vi "UE9 Stream Example LJ_swNONE.vi"() -> ()   [LabVIEW 2021]
panel:
  out "UD Backlog [%]":dbl format="%.2f"
  in  "AIN Range":u16(ring) items=["LJ_rgBIP5V", "LJ_rgUNI5V", "LJ_rgUNI2P5V", "LJ_rgUNI1P25V", "LJ_rgUNIP625V"]
  out "Actual Scan Rate (Hz)":dbl=1000.0 format="%.3f"
  out "ms Per Loop":u32
  out "Comm Backlog":dbl format="%.2f"
  out "Scans Retrieved Sec (measured)":dbl format="%.2f"
  out "# Scans Read":i32
  out "# of iterations":i32
  out "Data":dbl[][](array[numeric]) format="%.3f"
  in  "Scan Rate (Hz)":dbl=1000.0 format="%.3f"
  in  "Scan List":u8[](array[numeric])=[0, 1, 2, 3]
  in  "Data File Extension":string="dat"
  out "Current Data File":path
  in  "Data File Prefix":string="data"
  in  "Write To File":bool
  in  "FirstFound":bool=TRUE
  in  "stop":bool
  in  "ConnectionType":u16(ring) items=["LJ_ctUSB", "LJ_ctETHERNET"]
  in  "Address":string="192.168.1.209"
  out "Error Message":string
  in  "Resolution":i32=12
  # "The actual scans/sec is controlled\nby hardware and is known.  This\n\"measured\" suggests the rate at\nwhich data is being retreived."
  # "Specify an IP address for Ethernet, or Local ID\nfor USB.  If FirstFound is selected, Local ID is\nignored for USB.  Clear FirstFound if using Ethernet."
  # "(for all channels)"
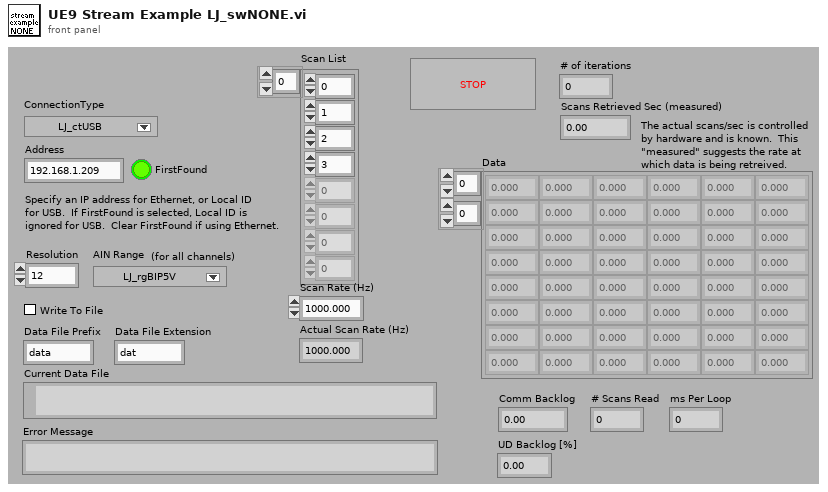
[diagram p1: front panel]
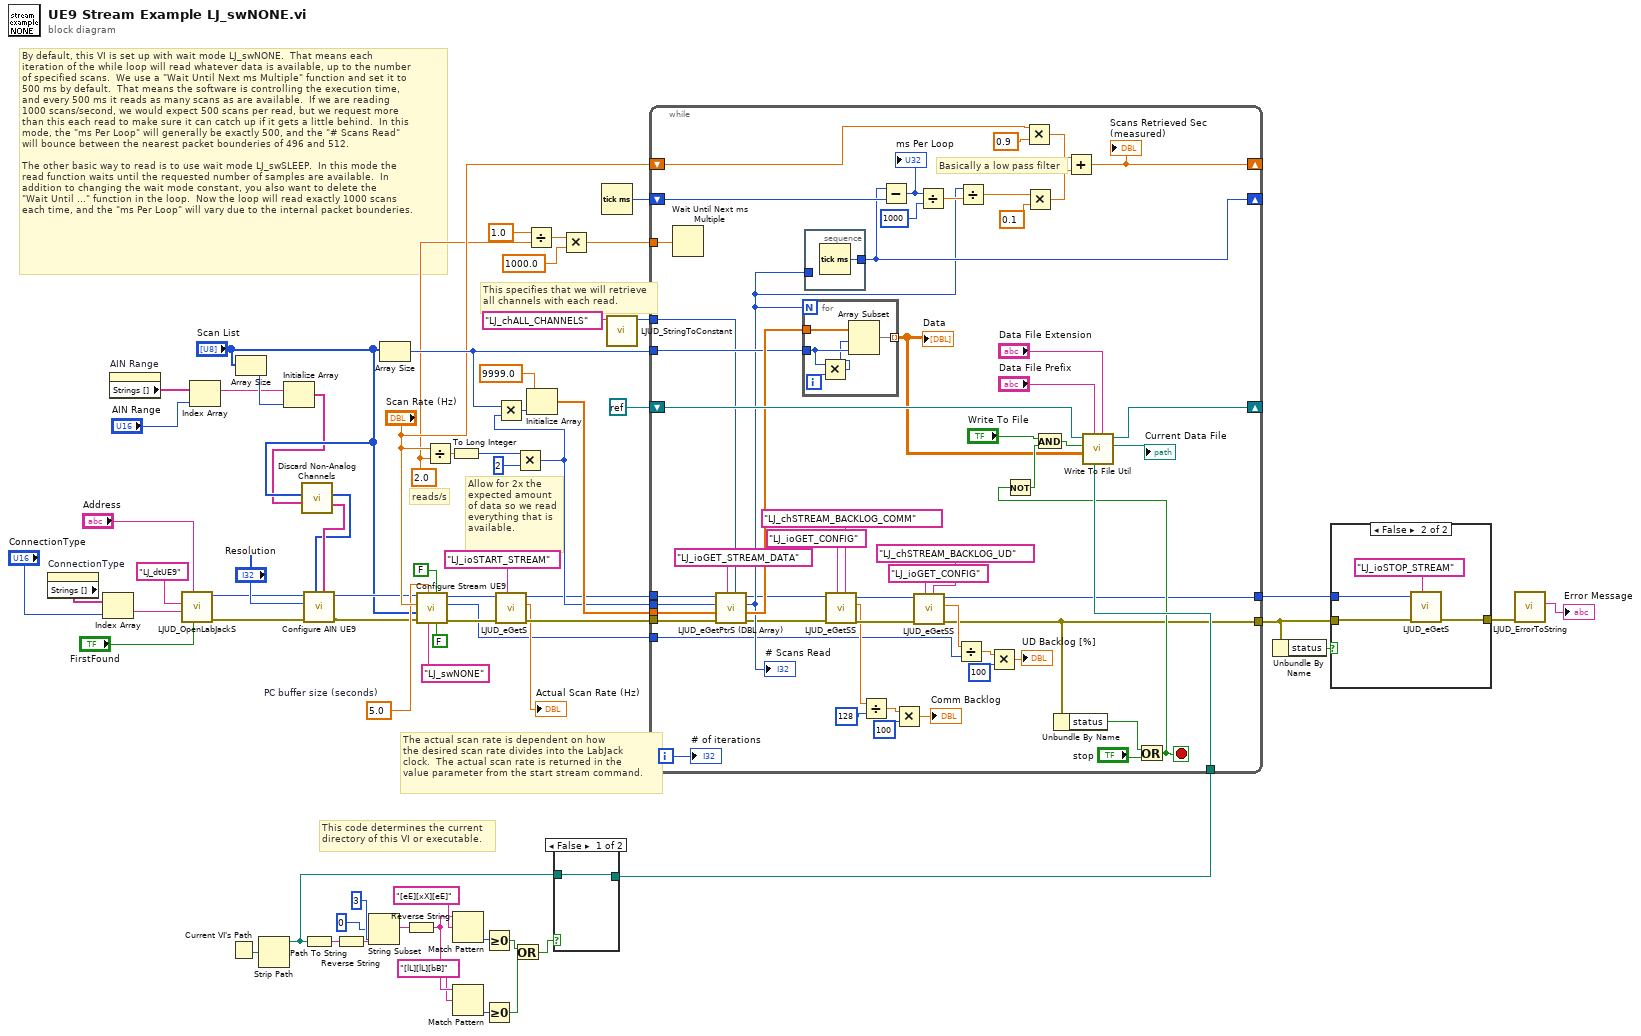
[diagram p0: block diagram]
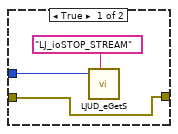
[diagram p2: hidden frame]
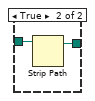
[diagram p3: hidden frame]
diagram:
  w30 = 5.0  # PC buffer size (seconds)
  w37 = 2.0 ("y")
  # "This specifies that we will retrieve\nall channels with each read."
  # "The actual scan rate is dependent on how\nthe desired scan rate divides into the LabJack\nclock.  The actual scan rate is returned in the\nvalue parameter from the start stream command."
  # "By default, this VI is set up with wait mode LJ_swNONE.  That means each\niteration of the while loop will read whatever data is available, up to the number\nof specified scans.  We use a \"Wait Until Next ms Multiple\" function and set it to\n500 ms by default.  That means the software is controlling the execution time,\nand every 500 ms it reads as many scans as are available.  If we are reading\n1000 scans/second, we would expect 500 scans per read, but we request more\nthan this each read to make sure it can catch up if it gets a little behind.  In this\nmode, the \"ms Per Loop\" will generally be exactly 500, and the \"# Scans Read\"\nwill bounce between the nearest packet bounderies of 496 and 512.\n\nThe other basic way to read is to use wait mode LJ_swSLEEP.  In this mode the\nread function waits until the requested number of samples are available.  In\naddition to changing the wait mode constant, you also want to delete the\n\"Wait Until ...\" function in the loop.  Now the loop will read exactly 1000 scans\neach time, and the \"ms Per Loop\" will vary due to the internal packet bounderies."
  # "reads/s"
  # "Allow for 2x the\nexpected amount\nof data so we read\neverything that is\navailable."
  # "This code determines the current\ndirectory of this VI or executable."
  n1 = property on="ConnectionType" class="Ring (strict)"() -> ("Strings []"=w12:string[])  [unwired: 2 in, 2 out]
  n2 = Index Array(array=w12, index="ConnectionType") -> (element=w10:string)
  n3 = property on="AIN Range" class="Ring (strict)"() -> ("Strings []"=w20:string[])  [unwired: 2 in, 2 out]
  n4 = call "LJUD_OpenLabJackS.vi"("FirstFound"="FirstFound", "Address"="Address", "ConnectionType"=w10, "DeviceType"="LJ_dtUE9") -> ("error out"=w16:errorcluster, "Handle"=w17:i32)  [unwired: 5 in, 1 out]
  n5 = Index Array(array=w20, index="AIN Range") -> (element=w18:string)
  n6 = Current VI's Path() -> (path=w68:path)
  n7 = Array Size(array="Scan List") -> (size(s)=w23:i32)
  n8 = Strip Path(path=w68) -> (stripped path=w60:path)  [unwired: 1 out]
  n9 = Initialize Array(w18, w23) -> (w4:string[])
  n10 = call "Discard Non-Analog Channels.vi"("Ranges In"=w4, "Channels In"="Scan List") -> ("Ranges Out"=w3:string[], "Channels Out"=w2:i32[])  [unwired: 6 in, 2 out]
  n11 = call "Configure AIN UE9.vi"("Ranges"=w3, "Channels"=w2, "error in"=w16, "Resolution"="Resolution", "Handle In"=w17) -> ("error out"=w26:errorcluster, "Handle Out"=w25:i32)  [unwired: 5 in]
  n12 = Path To String(path=w60) -> (string=w67:string)
  n13 = Reverse String(1:w67) -> (0:w66:string)
  n14 = String Subset(string=w66, offset (0)=0, length (rest)=3 ("length")) -> (substring=w63:string)
  n15 = Array Size(array="Scan List") -> (size(s)=w44:i32)
  n16 = Reverse String(1:w63) -> (0:w59:string)
  n17 = call "Configure Stream UE9.vi"("External Scan Trigger"=FALSE, "Scan Clock Output"=FALSE, "Wait Mode"="LJ_swNONE" ("Wait Mode (2)"), "PC buffer size (seconds)"=w30, "error in"=w26, "Scan List"="Scan List", "Scan Rate (Hz)"="Scan Rate (Hz)", "Handle In"=w25) -> ("error out"=w50:errorcluster, "PC buffer size (samples)"=w1:i32, "Handle Out"=w51:i32)  [unwired: 1 in]
  n18 = Divide(x="Scan Rate (Hz)", y=w37) -> (x/y=w48:dbl)
  n19 = To Long Integer(number=w48) -> (32bit integer=w33:i32)
  n20 = Match Pattern(string=w59, regular expression="[eE][xX][eE]") -> (offset past match=w61:i32)  [unwired: 1 in, 3 out]
  n21 = Match Pattern(string=w59, regular expression="[lL][lL][bB]") -> (offset past match=w56:i32)  [unwired: 1 in, 3 out]
  n22 = Greater Or Equal To 0?(x=w61) -> (x >= 0?=w57:bool)
  n23 = Greater Or Equal To 0?(x=w56) -> (x >= 0?=w55:bool)
  n24 = call "LJUD_eGetS.vi"("IOType"="LJ_ioSTART_STREAM", "error in"=w50, "Handle In"=w51) -> ("error out"=w49:errorcluster, "Value Read"=→"Actual Scan Rate (Hz)":dbl, "Handle Out"=w21:i32)  [unwired: 6 in]
  n25 = Or(x=w57, y=w55) -> (x .or. y?=w54:bool)
  n26 = Multiply(x=w33, y=2) -> (x*y=w32:i32)
  n27 = Multiply(x=w44, y=w32) -> (x*y=w47:i32)
  n28 = Divide(x=1.0, y=w37) -> (x/y=w35:dbl)
  n29 = Initialize Array(9999.0, w47) -> (w45:dbl[])
  n30 = case shown="False" w54 {
    tunnel: w60 -> [w70 w72]
    tunnel: [w70 w71] -> w53
    frame False {
    }
    frame True {
      n31 = Strip Path(path=w72) -> (stripped path=w71:path)  [unwired: 1 out]
    }
  }
  n32 = Multiply(x=w35, y=1000.0) -> (x*y=w22:dbl)
  n33 = Tick Count (ms)() -> (millisecond timer value=w39:u32)
  n34 = call "LJUD_StringToConstant.vi"("String"="LJ_chALL_CHANNELS") -> ("Constant Number"=w6:i32)  [unwired: 9 in, 1 out]
  n35 = while {
    tunnel: w1 -> [w73]
    tunnel: w6 -> [w89]
    tunnel: w22 -> [w90]
    shift-left: "Scan Rate (Hz)" -> [w98]
    shift-right: [w95] -> _
    shift-left: w39 -> [w107]
    shift-right: [w104] -> _
    tunnel: [w81] -> w8
    tunnel: [w79] -> w42
    tunnel: w44 -> [w110]
    tunnel: w45 -> [w113]
    tunnel: w32 -> [w111]
    tunnel: w53 -> [w118]
    shift-left: refnum<k0> refnum -> [w124]
    shift-right: [w123] -> _
    tunnel: w49 -> [w115]
    tunnel: w21 -> [w116]
    i -> [w108]
    stop <- w117 stop-if-true
    # "Basically a low pass filter"
    n36 = Wait Until Next ms Multiple(millisecond multiple=w90) -> ()  [unwired: 1 out]
    n37 = call "LJUD_eGetPtrS (DBL Array).vi"("Channel"=w89, "IOType"="LJ_ioGET_STREAM_DATA", "error in"=w115, "DBL Array Write"=w113, "Value"=w111, "Handle In"=w116) -> ("error out"=w93:errorcluster, "DBL Array Read"=w112:dbl[], "Value"=w102:i32, "Handle Out"=w94:i32)  [unwired: 2 in]
    "# Scans Read" <- w102
    n38 = for {
      N: w102 -> [_]
      tunnel: w112 -> [w134]
      tunnel: w110 -> [w133]
      tunnel: [w130] -> w109 mode=indexing
      i -> [w132]
      n39 = Multiply(x=w133, y=w132) -> (x*y=w131:i32)
      n40 = Array Subset(array=w134, index=w131, length=w133) -> (w130:dbl[])
    }
    "Data" <- w109
    n41 = stacked-sequence {
      tunnel: w102 -> [_]
      tunnel: [w129] -> w104
      frame #0 {
        n42 = Tick Count (ms)() -> (millisecond timer value=w129:u32)
      }
    }
    n43 = call "LJUD_eGetSS.vi"("Channel"="LJ_chSTREAM_BACKLOG_COMM", "IOType"="LJ_ioGET_CONFIG", "error in"=w93, "Handle In"=w94) -> ("error out"=w82:errorcluster, "Value Read"=w75:dbl, "Handle Out"=w83:i32)  [unwired: 5 in]
    n44 = Divide(x=w75, y=128) -> (x/y=w78:dbl)
    n45 = Subtract(x=w104, y=w107) -> (x-y=w106:u32)
    "ms Per Loop" <- w106
    n46 = Multiply(x=w78, y=100) -> (x*y=→"Comm Backlog":dbl)
    n47 = call "LJUD_eGetSS.vi"("Channel"="LJ_chSTREAM_BACKLOG_UD", "IOType"="LJ_ioGET_CONFIG", "error in"=w82, "Handle In"=w83) -> ("error out"=w81:errorcluster, "Value Read"=w84:dbl, "Handle Out"=w79:i32)  [unwired: 5 in]
    n48 = Divide(x=w106, y=u32 1000) -> (x/y=w103:dbl)
    n49 = Divide(x=w84, y=w73) -> (x/y=w85:dbl)
    n50 = Divide(x=w102, y=w103) -> (x/y=w101:dbl)
    n51 = Multiply(x=w85, y=100) -> (x*y=→"UD Backlog [%]":dbl)
    n52 = Multiply(x=w98, y=0.9) -> (x*y=w97:dbl)
    n53 = Multiply(x=w101, y=0.1) -> (x*y=w96:dbl)
    n54 = Unbundle By Name(w81) -> ("status"=w127:bool)
    n55 = Add(x=w97, y=w96) -> (x+y=w95:dbl)
    "Scans Retrieved Sec (measured)" <- w95
    n56 = Or(x=w127, y="stop") -> (x .or. y?=w117:bool)
    n57 = Not(x=w117) -> (.not. x?=w119:bool)
    n58 = And(x="Write To File", y=w119) -> (x .and. y?=w120:bool)
    n59 = call "Write To File Util.vi"("Data File Extension"="Data File Extension", "Working Directory"=w118, "Data File Prefix"="Data File Prefix", "Data"=w109, "Write To File"=w120, "File Refnum In"=w124) -> ("Current Data File"=→"Current Data File":path, "File Refnum Out"=w123:refnum<file>)  [unwired: 3 in, 1 out]
    "# of iterations" <- w108
  }
  n60 = Unbundle By Name(w8) -> ("status"=w9:bool)
  n61 = case shown="False" w9 {
    tunnel: w42 -> [w136 w140]
    tunnel: [w135 w139] -> w41
    tunnel: w8 -> [w135 w138]
    frame True {
      n62 = call "LJUD_eGetS.vi"("IOType"="LJ_ioSTOP_STREAM", "Handle In"=w136) -> ()  [unwired: 7 in, 3 out]
    }
    frame False {
      n63 = call "LJUD_eGetS.vi"("IOType"="LJ_ioSTOP_STREAM", "error in"=w138, "Handle In"=w140) -> ("error out"=w139:errorcluster)  [unwired: 6 in, 2 out]
    }
  }
  n64 = call "LJUD_ErrorToString.vi"("error in"=w41) -> ("String"=→"Error Message":string)  [unwired: 10 in]
